vi "ClientNetworkInterface.vi"() -> ()   [LabVIEW 2025]
uses:
  <vilib>/net/WFCN/Network Status.ctl
  ClientNetworkInterfaceGlobalVariables.vi
  <vilib>/net/WFCN/NI_WFCN.lvlib
panel:
  out "error out":errorcluster
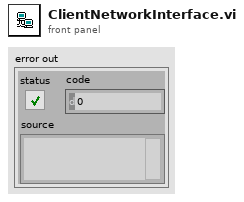
[diagram p1: front panel]
types:
  T1 = typedef "NI_WFCN.lvlib/Network Status.ctl" = enum16{"Indeterminate", "Configured", "Unconfigured"}
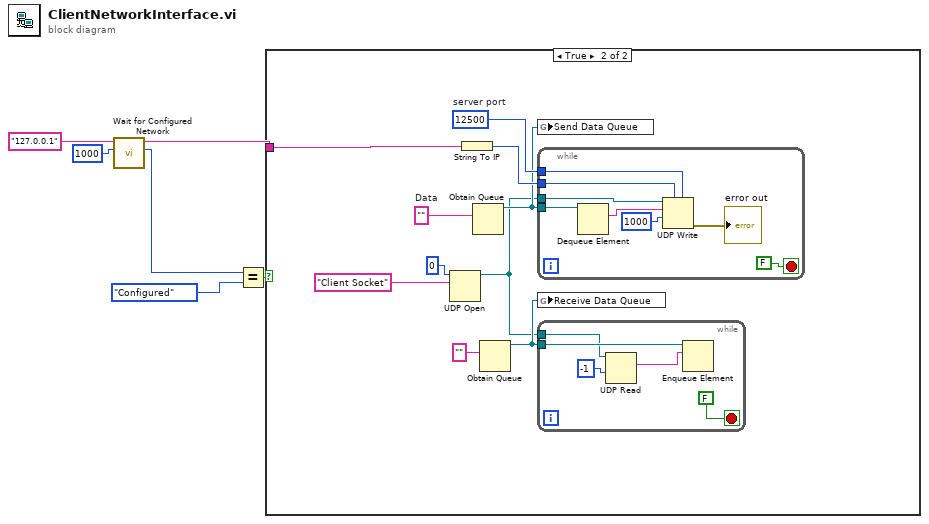
[diagram p0: block diagram]
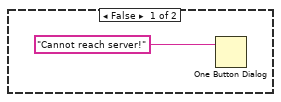
[diagram p2: hidden frame]
diagram:
  n1 = call <vilib>:"Wait for Configured Network.vi"("timeout in ms"=1000, "hostname or URL in"="127.0.0.1" ("name")) -> ("network status for remote host"=w2:T1, "hostname or URL out"=w4:string)  [unwired: 8 in]
  n2 = Equal?(x=w2, y=Network_Status."Configured" ("network status for remote host")) -> (x = y?=w3:bool)
  n3 = case shown="True" w3 {
    tunnel: w4 -> [_ w11]
    frame False {
      n4 = One Button Dialog(message="Cannot reach server!") -> ()  [unwired: 1 in, 1 out]
    }
    frame True {
      w15 = u16 12500  # server port
      w16 = ""  # Data
      n5 = UDP Open(10:"Client Socket" ("service name"), 11:u16 0 ("port")) -> (port=w8:refnum<k16>)  [unwired: 3 in, 2 out]
      n6 = String To IP(1:w11) -> (0:w14:u32)
      n7 = Obtain Queue(element data type=w16) -> (queue out=w12:refnum<queue>)  [unwired: 4 in, 2 out]
      n8 = Obtain Queue(element data type="") -> (queue out=w13:refnum<queue>)  [unwired: 4 in, 2 out]
      n9 = global write "ClientNetworkInterfaceGlobalVariables.vi" "Send Data Queue"(w12) -> ()
      n10 = while {
        tunnel: w12 -> [w25]
        tunnel: w14 -> [w22]
        tunnel: w15 -> [w21]
        tunnel: w8 -> [w18]
        stop <- FALSE stop-if-true
        n11 = Dequeue Element(queue=w25) -> (element=w24:string)  [unwired: 2 in, 3 out]
        n12 = UDP Write(address=w22, port or service name=w21, connection ID=w18, data in=w24, 9:1000 ("timeout ms (25000)")) -> (error out=→"error out":errorcluster)  [unwired: 1 in, 1 out]
      }
      n13 = global write "ClientNetworkInterfaceGlobalVariables.vi" "Receive Data Queue"(w13) -> ()
      n14 = while {
        tunnel: w13 -> [w30]
        tunnel: w8 -> [w26]
        stop <- FALSE stop-if-true
        n15 = UDP Read(connection ID=w26, timeout ms (25000)=-1) -> (data out=w29:string)  [unwired: 2 in, 4 out]
        n16 = Enqueue Element(queue=w30, element=w29) -> ()  [unwired: 2 in, 3 out]
      }
    }
  }
